vi "RunTestSuite.vi"(8 "error in":errorcluster) -> (0 "error out":errorcluster)   [LabVIEW 2020, in "CICD.lvlib"]
uses:
  CICD.lvlib
  <vilib>/Wiresmith Technology/G CLI/Argument Parser/Option Class/Option Configuration.ctl
  <vilib>/Wiresmith Technology/G CLI/Argument Parser/Option Class/Argument Type.ctl
  <vilib>/Wiresmith Technology/G CLI/CLI Class/CLI.lvclass
  <vilib>/Wiresmith Technology/G CLI/Argument Parser/Option Set Class/Option Set.lvclass
  <vilib>/Wiresmith Technology/G CLI/Argument Parser/Option Class/Option.lvclass
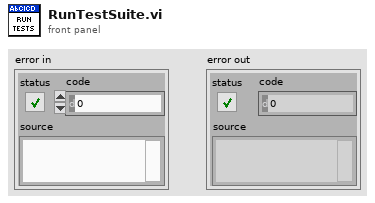
[diagram p1: front panel]
types:
  T1 = typedef "Option Parser.lvlib/Option.lvclass/Option Configuration.ctl" = cluster{"Option Type":T2, "Option Labels":string[], "Key":string, "Description":string, "Required":bool, "Default Value":string}
  T2 = typedef "Option Parser.lvlib/Option.lvclass/Argument Type.ctl" = enum16{"flag", "value"}
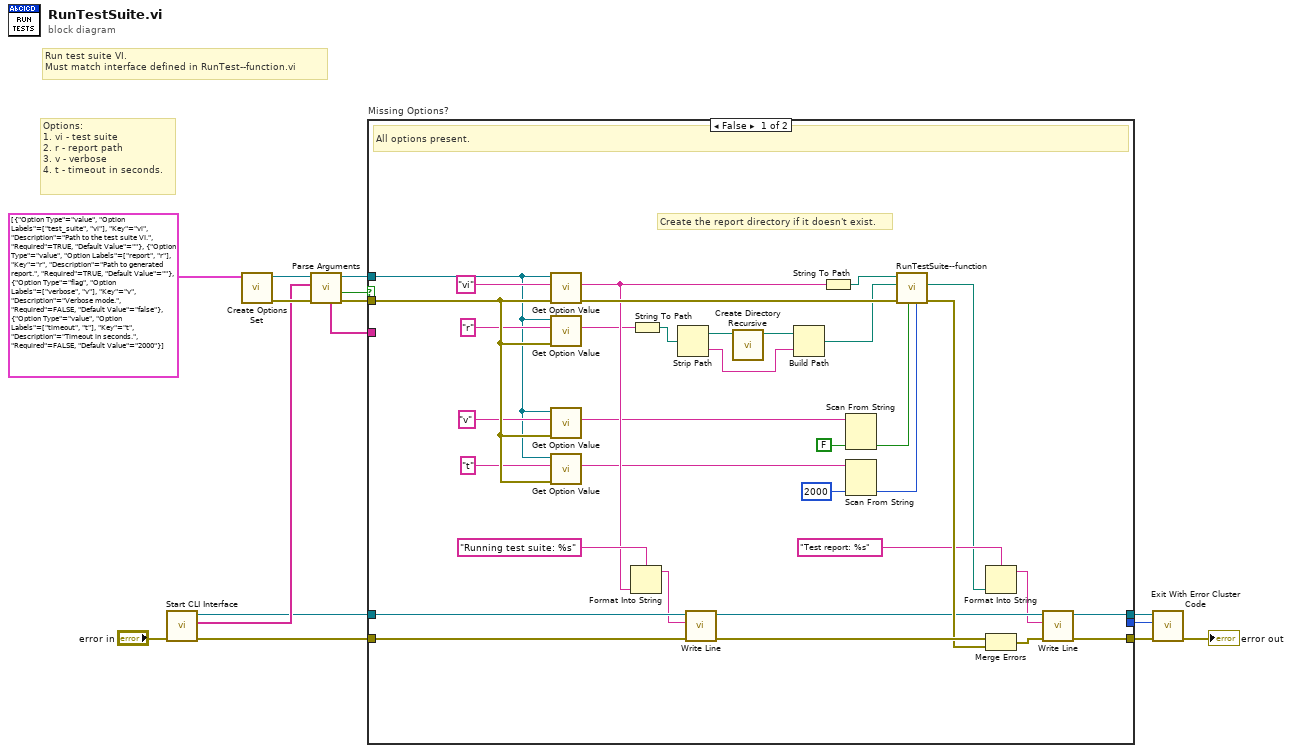
[diagram p0: block diagram]
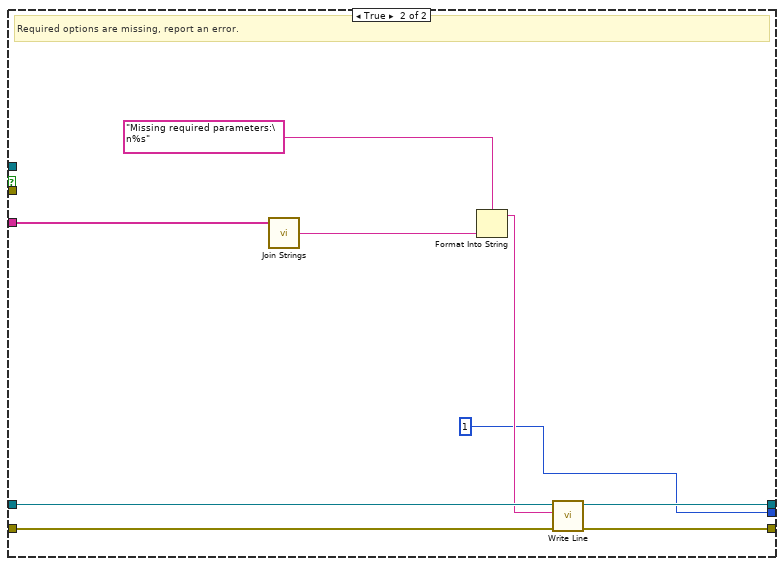
[diagram p2: hidden frame]
diagram:
  # "Run test suite VI.\nMust match interface defined in RunTest--function.vi"
  # "Options:\n1. vi - test suite\n2. r - report path\n3. v - verbose\n4. t - timeout in seconds."
  n1 = call <vilib>:"Start CLI Interface.vi"("error in (no error)"="error in") -> ("error out"=w12:errorcluster, "Custom Parameters"=w8:string[], "CLI out"=w5:refnum<class "CLI.lvclass">)  [unwired: 7 in, 1 out]
  n2 = call <vilib>:"Create Options Set.vi"("Options"=T1[] [{"Option Type"=enum."value", "Option Labels"=["test_suite", "vi"], "Key"="vi", "Description"="Path to the test suite VI.", "Required"=TRUE, "Default Value"=""}, {"Option Type"=enum."value", "Option Labels"=["report", "r"], "Key"="r", "Description"="Path to generated report.", "Required"=TRUE, "Default Value"=""}, {"Option Type"=enum."flag", "Option Labels"=["verbose", "v"], "Key"="v", "Description"="Verbose mode.", "Required"=FALSE, "Default Value"="false"}, {"Option Type"=enum."value", "Option Labels"=["timeout", "t"], "Key"="t", "Description"="Timeout in seconds.", "Required"=FALSE, "Default Value"="2000"}]) -> ("error out"=w14:errorcluster, "Option Set out"=w9:refnum<class "Option Set.lvclass">)  [unwired: 9 in]
  n3 = call <vilib>:"Parse Arguments.vi"("error in (no error)"=w14, "Arguments"=w8, "Option Set in"=w9) -> ("error out"=w13:errorcluster, "Missing Options"=w7:bool, "Option Set out"=w2:refnum<class "Option Set.lvclass">, "Missing Option Keys"=w6:string[])  [unwired: 5 in]
  n4 = case "Missing Options?" shown="False" w7 {
    tunnel: w13 -> [w46 _]
    tunnel: w6 -> [_ w54]
    tunnel: w12 -> [w49 w58]
    tunnel: w5 -> [w41 w53]
    tunnel: [w45 w57] -> w11
    tunnel: [w25 w51] -> w4
    tunnel: [_ 1 ("No Error Code (0)")] -> w3
    tunnel: w2 -> [w35 _]
    frame False {
      # "Create the report directory if it doesn't exist."
      # "All options present."
      n5 = call <vilib>:"Get Option Value.vi"("error in (no error)"=w46, "Option Key"="vi", "Option Set in"=w35) -> ("error out"=w47:errorcluster, "Value"=w34:string)  [unwired: 5 in, 2 out]
      n6 = call <vilib>:"Get Option Value.vi"("error in (no error)"=w46, "Option Key"="r", "Option Set in"=w35) -> ("Value"=w32:string)  [unwired: 5 in, 3 out]
      n7 = call <vilib>:"Get Option Value.vi"("error in (no error)"=w46, "Option Key"="v", "Option Set in"=w35) -> ("Value"=w29:string)  [unwired: 5 in, 3 out]
      n8 = call <vilib>:"Get Option Value.vi"("error in (no error)"=w46, "Option Key"="t", "Option Set in"=w35) -> ("Value"=w27:string)  [unwired: 5 in, 3 out]
      n9 = Format Into String(format string="Running test suite: %s", w34) -> (resulting string=w39:string)  [unwired: 2 in, 1 out]
      n10 = String To Path(string=w32) -> (path=w20:path)
      n11 = Strip Path(path=w20) -> (stripped path=w19:path, name=w17:string)
      n12 = call <vilib>:"Write Line.vi"("error in (no error)"=w49, "Text to Write"=w39, "CLI in"=w41) -> ("error out"=w48:errorcluster, "CLI out"=w24:refnum<class "CLI.lvclass">)  [unwired: 7 in]
      n13 = call <vilib>:"Create Directory Recursive.vi"("directory"=w19) -> ("directory copy"=w18:path)  [unwired: 4 in, 2 out]
      n14 = Build Path(base path=w18, name or relative path=w17) -> (appended path=w16:path)
      n15 = String To Path(string=w34) -> (path=w33:path)
      n16 = Scan From String(input string=w29, default 1=FALSE) -> (output 1=w30:bool)  [unwired: 3 in, 3 out]
      n17 = Scan From String(input string=w27, default 1=2000) -> (output 1=w26:i32)  [unwired: 3 in, 3 out]
      n18 = call "RunTestSuite--function.vi"("timeout (s) (2000)"=w26, "Verbose (F)"=w30, "error in"=w47, "Report Path"=w16, "Test Suite (.vi)"=w33) -> ("error out"=w43:errorcluster, "Report Path"=w22:path)  [unwired: 4 in, 1 out]
      n19 = Format Into String(format string="Test report: %s", w22) -> (resulting string=w21:string)  [unwired: 2 in, 1 out]
      n20 = Merge Errors(w48, w43) -> (w44:errorcluster)
      n21 = call <vilib>:"Write Line.vi"("error in (no error)"=w44, "Text to Write"=w21, "CLI in"=w24) -> ("error out"=w45:errorcluster, "CLI out"=w25:refnum<class "CLI.lvclass">)  [unwired: 7 in]
    }
    frame True {
      # "Required options are missing, report an error."
      n22 = call <vilib>:"Join Strings.vi"("Strings In"=w54) -> ("String"=w55:string)  [unwired: 2 in]
      n23 = Format Into String(format string="Missing required parameters:\n%s" ("Text to Write"), w55) -> (resulting string=w52:string)  [unwired: 2 in, 1 out]
      n24 = call <vilib>:"Write Line.vi"("error in (no error)"=w58, "Text to Write"=w52, "CLI in"=w53) -> ("error out"=w57:errorcluster, "CLI out"=w51:refnum<class "CLI.lvclass">)  [unwired: 7 in]
    }
  }
  n25 = call <vilib>:"Exit With Error Cluster Code.vi"("error in (no error)"=w11, "No Error Code (0)"=w3, "CLI in"=w4) -> ("error out"=→"error out":errorcluster)  [unwired: 8 in]
